vi "Get 1D DBL Q on Variant.vi"(8 "error in (no error)":errorcluster, 11 "Variant in":variant) -> (0 "error out":errorcluster, 1 "1d DBL Data Queue":T1, 3 "Variant out":variant)   [LabVIEW 2020, in "Internal Comm Classes.lvlib" / "WPL Comm (1D DBL).lvclass"]
uses:
  WPL Comm (1D DBL).lvclass
  Waveform 1d dbl queue.ctl
  <vilib>/Utility/error.llb/Error Cluster From Error Code.vi
  WPL Comm.lvclass
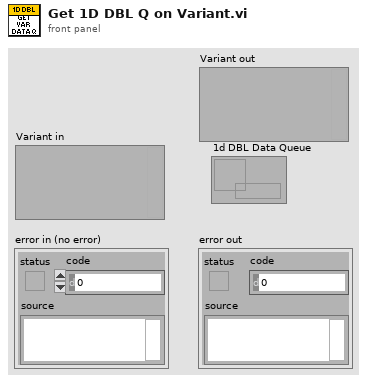
[diagram p1: front panel]
types:
  T1 = typedef "Internal Comm Classes.lvlib/WPL Comm (1D DBL).lvclass/Waveform 1d dbl queue.ctl" = refnum<queue>
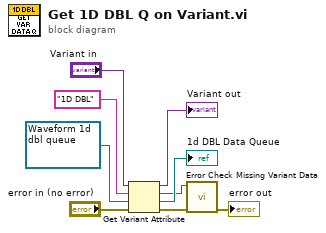
[diagram p0: block diagram]
diagram:
  n1 = Get Variant Attribute(Variant="Variant in", name="1D DBL", default value (empty Variant)=T1 refnum ("Queue in"), error in="error in (no error)") -> (duplicate Variant=→"Variant out":variant, found=w3:bool, value=→"1d DBL Data Queue":T1, error out=w2:errorcluster)
  n2 = call "Error Check Missing Variant Data.vi"("error in (no error)"=w2, "Found?"=w3) -> ("error out"=→"error out":errorcluster)  [unwired: 9 in]
